vi "array -- get segment.vi"(4 "max T":dbl=nan, 6 "min T":dbl=nan, 10 "other points":dbl[](array[numeric]), 11 "temperature points":dbl[](array[numeric])) -> (2 "other segment":dbl[](array[numeric]))   [LabVIEW 2014]
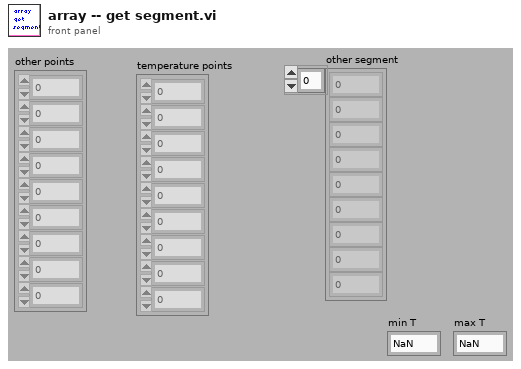
[diagram p1: front panel]
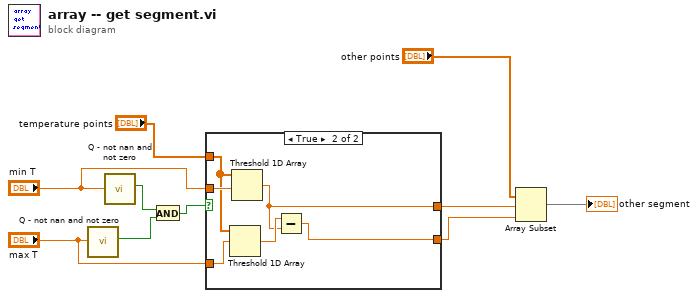
[diagram p0: block diagram]
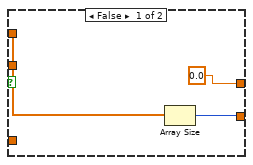
[diagram p2: hidden frame]
diagram:
  n1 = call "Q - not nan and not zero.vi"("Numeric"="max T") -> ("Boolean"=w9:bool)  [unwired: 10 in]
  n2 = call "Q - not nan and not zero.vi"("Numeric"="min T") -> ("Boolean"=w10:bool)  [unwired: 10 in]
  n3 = And(x=w10, y=w9) -> (x .and. y?=w6:bool)
  n4 = case shown="True" w6 {
    tunnel: "min T" -> [_ w19]
    tunnel: "max T" -> [_ w18]
    tunnel: [0.0 w16] -> w5
    tunnel: [w13 w15] -> w4
    tunnel: "temperature points" -> [w11 w14]
    frame False {
      n5 = Array Size(array=w11) -> (size(s)=w13:i32)
    }
    frame True {
      n6 = Threshold 1D Array(2:w18, 3:w14) -> (0:w17:dbl)  [unwired: 1 in]
      n7 = Threshold 1D Array(2:w19, 3:w14) -> (0:w16:dbl)  [unwired: 1 in]
      n8 = Subtract(x=w17, y=w16) -> (x-y=w15:dbl)
    }
  }
  n9 = Array Subset(array="other points", index=w5, length=w4) -> (→"other segment":dbl[])
